vi "Read Key (String).vi"(6 "Read Raw String? (F)":bool, 7 "Section Name":string, 8 "error in (no error)":errorcluster, 9 "Default":string, 10 "Key Name":string, 11 "Config in":refnum<class "LabVIEW-Config.lvclass">) -> (0 "error out":errorcluster, 1 "Value":string, 2 "Key Found?":bool, 3 "Config out":refnum<class "LabVIEW-Config.lvclass">)   [LabVIEW 2017, in "LabVIEW-Config.lvlib" / "LabVIEW-Config.lvclass"]
uses:
  LabVIEW-Config.lvclass
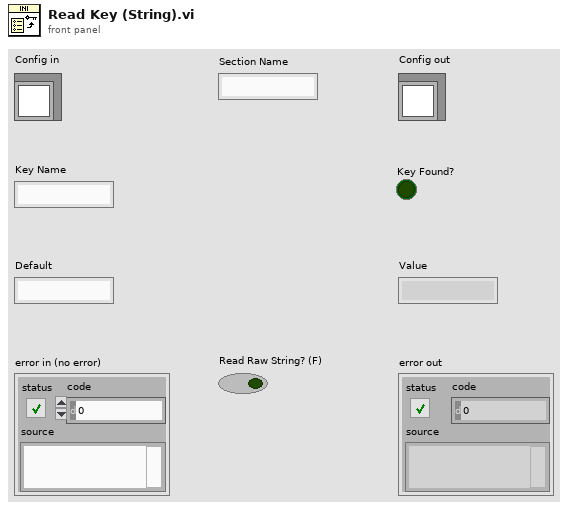
[diagram p1: front panel]
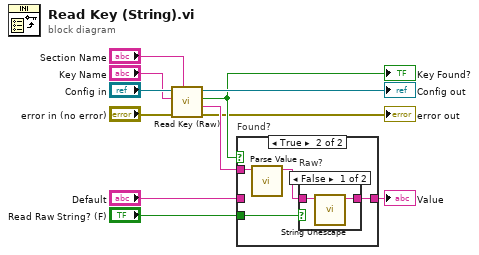
[diagram p0: block diagram]
diagram:
  n1 = call "Read Key (Raw).vi"("Section Name"="Section Name", "error in (no error)"="error in (no error)", "Key Name"="Key Name", "Config in"="Config in") -> ("error out"=→"error out":errorcluster, "Content"=w6:string, "Key Found?"=w5:bool, "Config out"=→"Config out":refnum<class "LabVIEW-Config.lvclass">)  [unwired: 4 in]
  "Key Found?" <- w5
  n2 = case "Found?" shown="True" w5 {
    tunnel: w6 -> [_ w16]
    tunnel: [w12 w14] -> w3
    tunnel: "Default" -> [w12 _]
    tunnel: "Read Raw String? (F)" -> [_ w13]
    frame False {
    }
    frame True {
      n3 = call "Parse Value.vi"("Value"=w16) -> ("Value (Quotes Removed)"=w15:string)  [unwired: 9 in, 1 out]
      n4 = case "Raw?" shown="False" w13 {
        tunnel: w15 -> [w18 w19]
        tunnel: [w17 w19] -> w14
        frame False {
          n5 = call "String Unescape.vi"("Escaped String"=w18) -> ("Unescaped String"=w17:string)  [unwired: 10 in]
        }
        frame True {
        }
      }
    }
  }
  "Value" <- w3
